vi "FTW-JSON-LexicalScan-Value.vi"(0 "JSON String":T1, 11 "error in":errorcluster) -> (4 "JSON String Out":T1, 8 "Container":variant, 15 "error out":errorcluster)   [LabVIEW 2015]
uses:
  FTW-JSON-LexicalScan.ctl
  container/FTW-Container.lvclass
panel:
  # "Inputs"
  # "Outputs"
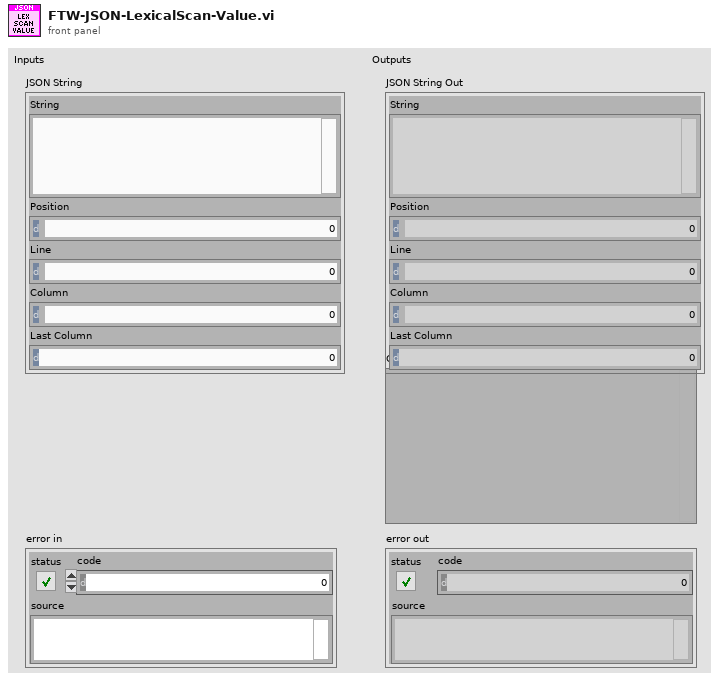
[diagram p1: front panel]
types:
  T1 = typedef "FTW-JSON-LexicalScan.ctl" = cluster{"String":string, "Position":i32, "Line":i32, "Column":i32, "Last Column":i32}
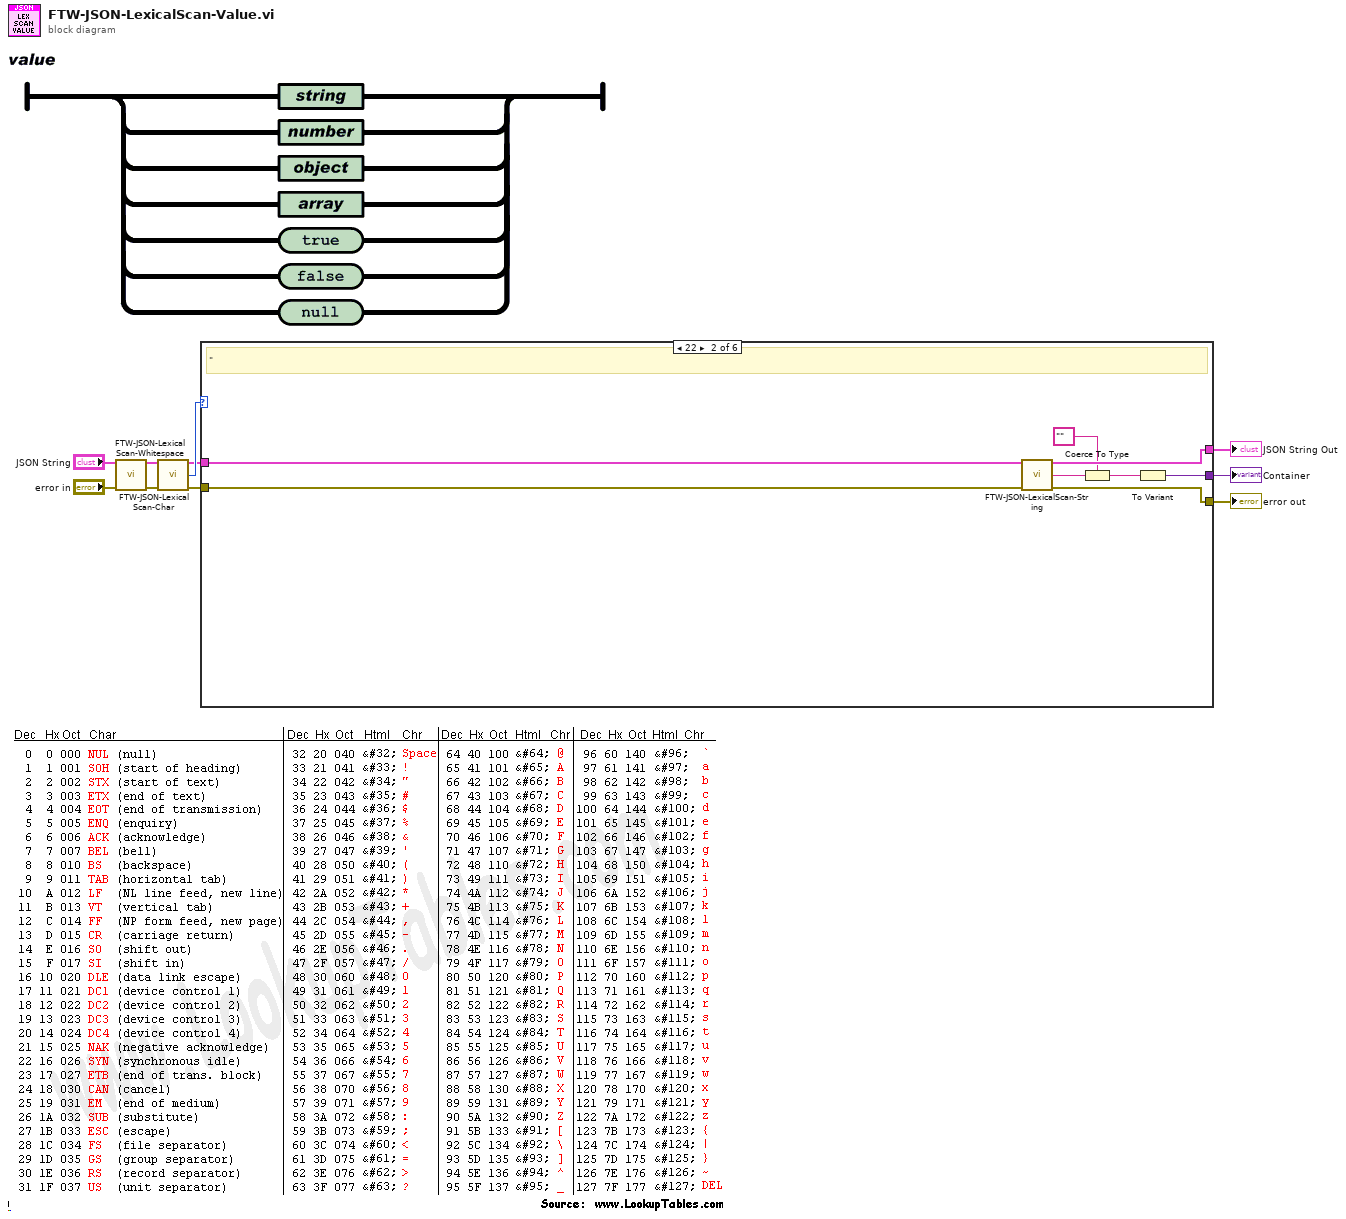
[diagram p0: block diagram]
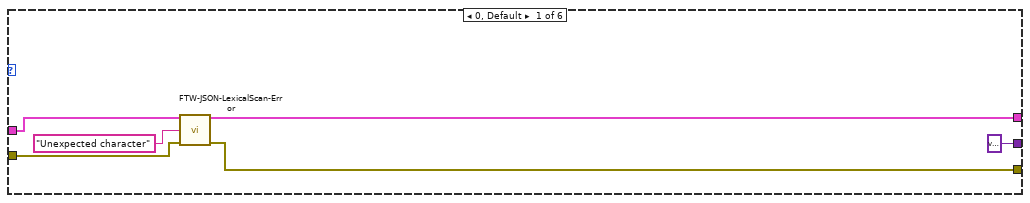
[diagram p2: hidden frame]
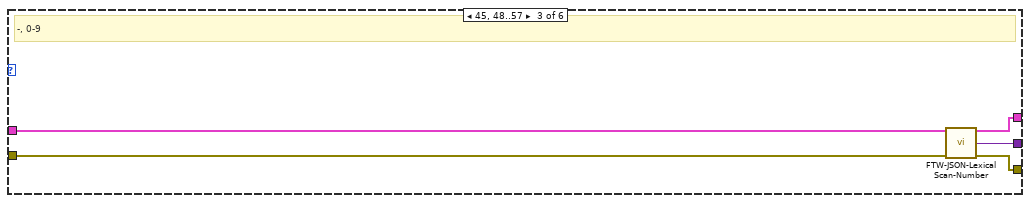
[diagram p3: hidden frame]
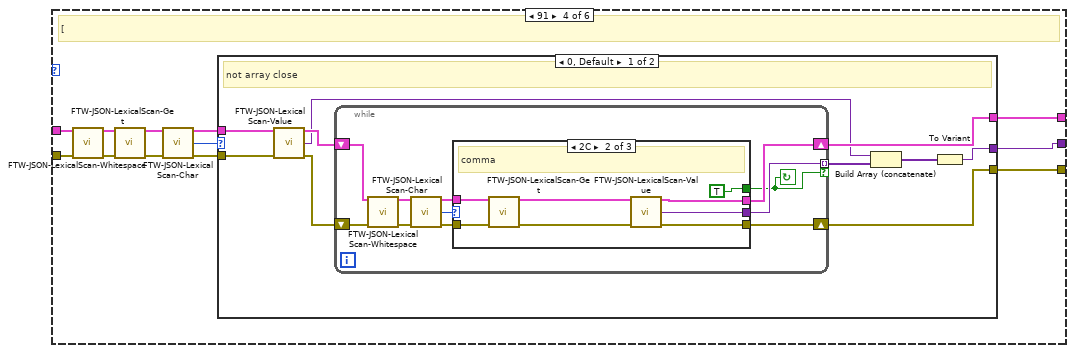
[diagram p4: hidden frame]
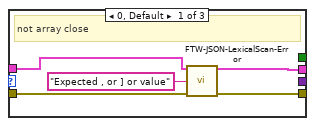
[diagram p5: hidden frame]
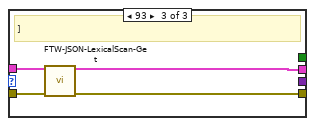
[diagram p6: hidden frame]
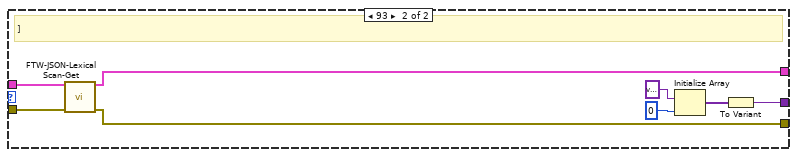
[diagram p7: hidden frame]
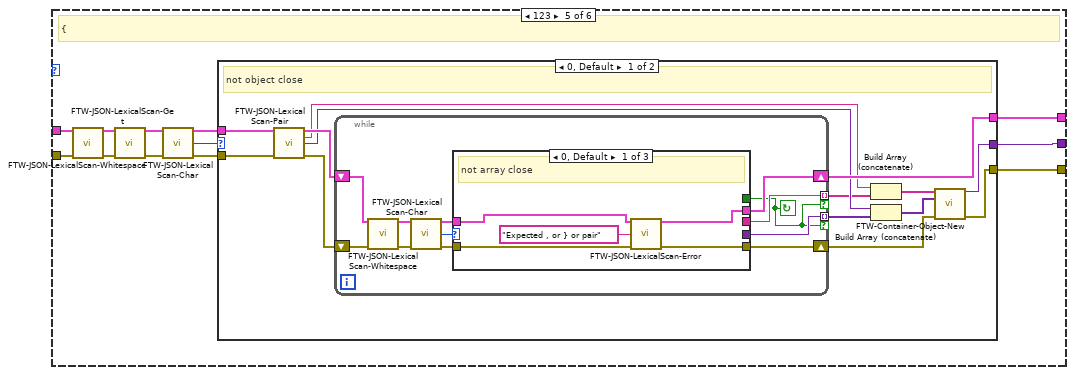
[diagram p8: hidden frame]
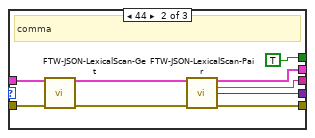
[diagram p9: hidden frame]
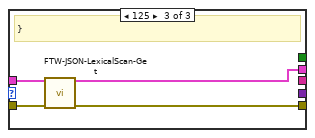
[diagram p10: hidden frame]
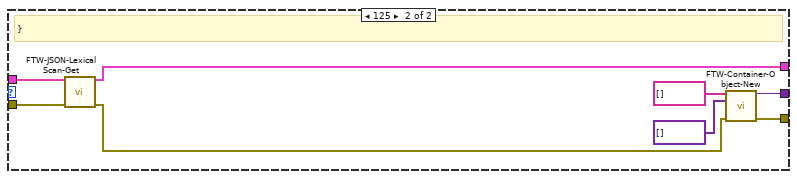
[diagram p11: hidden frame]
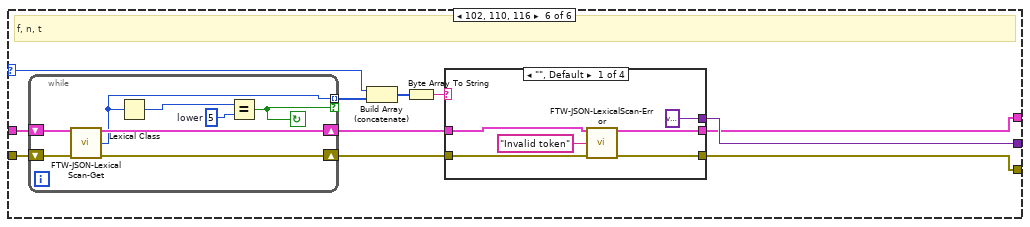
[diagram p12: hidden frame]
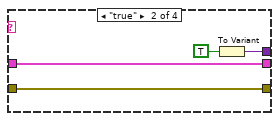
[diagram p13: hidden frame]
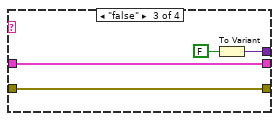
[diagram p14: hidden frame]
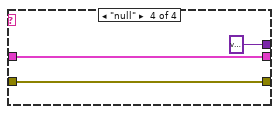
[diagram p15: hidden frame]
diagram:
  n1 = call "FTW-JSON-LexicalScan-Whitespace.vi"("JSON String"="JSON String", "error in"="error in") -> ("JSON String Out"=w1:T1, "error out"=w3:errorcluster)  [unwired: 12 in]
  n2 = call "FTW-JSON-LexicalScan-Char.vi"("JSON String"=w1, "error in"=w3) -> ("JSON String Out"=w7:T1, "Char"=w9:u8, "error out"=w8:errorcluster)  [unwired: 11 in]
  n3 = case shown="22" w9 {
    selector: w9 -> [_ _ _ _ _ w158]
    tunnel: w8 -> [w16 w23 w28 w41 w99 w161]
    tunnel: w7 -> [w13 w24 w29 w39 w97 w160]
    tunnel: [w14 w22 w27 w31 w89 w156] -> w6
    tunnel: [w12 w21 w26 w32 w90 w152] -> w5
    tunnel: [variant w19 w25 w30 w88 w154] -> w4
    frame 0, Default {
      n4 = call "FTW-JSON-LexicalScan-Error.vi"("JSON String"=w13, "Error String"="Unexpected character", "error in"=w16) -> ("JSON String Out"=w12:T1, "error out"=w14:errorcluster)  [unwired: 11 in]
    }
    frame 34 {
      # "\""
      n5 = call "FTW-JSON-LexicalScan-String.vi"("JSON String"=w24, "error in"=w23) -> ("JSON String Out"=w21:T1, "String"=w20:string, "error out"=w22:errorcluster)  [unwired: 10 in, 1 out]
      n6 = Coerce To Type(0:w20, 1:"") -> (2:w18:string)
      n7 = To Variant(anything=w18) -> (Variant=w19:variant)
    }
    frame 45, 48..57 {
      # "-, 0-9"
      n8 = call "FTW-JSON-LexicalScan-Number.vi"("JSON String"=w29, "error in"=w28) -> ("JSON String Out"=w26:T1, "Number"=w25:variant, "error out"=w27:errorcluster)  [unwired: 11 in]
    }
    frame 91 {
      # "["
      n9 = call "FTW-JSON-LexicalScan-Get.vi"("JSON String"=w39, "error in"=w41) -> ("JSON String Out"=w38:T1, "error out"=w40:errorcluster)  [unwired: 11 in, 1 out]
      n10 = call "FTW-JSON-LexicalScan-Whitespace.vi"("JSON String"=w38, "error in"=w40) -> ("JSON String Out"=w37:T1, "error out"=w36:errorcluster)  [unwired: 12 in]
      n11 = call "FTW-JSON-LexicalScan-Char.vi"("JSON String"=w37, "error in"=w36) -> ("JSON String Out"=w34:T1, "Char"=w35:u8, "error out"=w33:errorcluster)  [unwired: 11 in]
      n12 = case shown="0, Default" w35 {
        tunnel: w34 -> [w50 w81]
        tunnel: w33 -> [w51 w87]
        tunnel: [w46 w80] -> w32
        tunnel: [w47 w82] -> w31
        tunnel: [w42 w83] -> w30
        frame 0, Default {
          # "not array close"
          n13 = call "FTW-JSON-LexicalScan-Value.vi"("JSON String"=w50, "error in"=w51) -> ("JSON String Out"=w48:T1, "Container"=w44:variant, "error out"=w49:errorcluster)  [unwired: 11 in]
          n14 = while {
            shift-right: [w54] -> w47
            shift-left: w49 -> [w62]
            shift-right: [w55] -> w46
            shift-left: w48 -> [w60]
            tunnel: [w53] -> w45 mode=indexing if=w52
            stop <- w52 continue-if-true
            n15 = call "FTW-JSON-LexicalScan-Whitespace.vi"("JSON String"=w60, "error in"=w62) -> ("JSON String Out"=w59:T1, "error out"=w61:errorcluster)  [unwired: 12 in]
            n16 = call "FTW-JSON-LexicalScan-Char.vi"("JSON String"=w59, "error in"=w61) -> ("JSON String Out"=w58:T1, "Char"=w56:u8, "error out"=w57:errorcluster)  [unwired: 11 in]
            n17 = case shown="2C" w56 {
              tunnel: w58 -> [w65 w71 w77]
              tunnel: w57 -> [w67 w75 w79]
              tunnel: [w64 w73 w76] -> w55
              tunnel: [w66 w74 w78] -> w54
              tunnel: [_ w69 _] -> w53
              tunnel: [_ TRUE _] -> w52
              frame 0, Default {
                # "not array close"
                n18 = call "FTW-JSON-LexicalScan-Error.vi"("JSON String"=w65, "Error String"="Expected , or ] or value" ("Error Message"), "error in"=w67) -> ("JSON String Out"=w64:T1, "error out"=w66:errorcluster)  [unwired: 11 in]
              }
              frame 44 {
                # "comma"
                n19 = call "FTW-JSON-LexicalScan-Get.vi"("JSON String"=w71, "error in"=w75) -> ("JSON String Out"=w70:T1, "error out"=w72:errorcluster)  [unwired: 11 in, 1 out]
                n20 = call "FTW-JSON-LexicalScan-Value.vi"("JSON String"=w70, "error in"=w72) -> ("JSON String Out"=w73:T1, "Container"=w69:variant, "error out"=w74:errorcluster)  [unwired: 11 in]
              }
              frame 93 {
                # "]"
                n21 = call "FTW-JSON-LexicalScan-Get.vi"("JSON String"=w77, "error in"=w79) -> ("JSON String Out"=w76:T1, "error out"=w78:errorcluster)  [unwired: 11 in, 1 out]
              }
            }
          }
          n22 = Build Array (concatenate)(w44, w45) -> (w43:variant[])
          n23 = To Variant(anything=w43) -> (Variant=w42:variant)
        }
        frame 93 {
          # "]"
          n24 = call "FTW-JSON-LexicalScan-Get.vi"("JSON String"=w81, "error in"=w87) -> ("JSON String Out"=w80:T1, "error out"=w82:errorcluster)  [unwired: 11 in, 1 out]
          n25 = Initialize Array(variant, 0 ("dimension size")) -> (w84:variant[])
          n26 = To Variant(anything=w84) -> (Variant=w83:variant)
        }
      }
    }
    frame 123 {
      # "{"
      n27 = call "FTW-JSON-LexicalScan-Get.vi"("JSON String"=w97, "error in"=w99) -> ("JSON String Out"=w96:T1, "error out"=w98:errorcluster)  [unwired: 11 in, 1 out]
      n28 = call "FTW-JSON-LexicalScan-Whitespace.vi"("JSON String"=w96, "error in"=w98) -> ("JSON String Out"=w95:T1, "error out"=w94:errorcluster)  [unwired: 12 in]
      n29 = call "FTW-JSON-LexicalScan-Char.vi"("JSON String"=w95, "error in"=w94) -> ("JSON String Out"=w92:T1, "Char"=w93:u8, "error out"=w91:errorcluster)  [unwired: 11 in]
      n30 = case shown="0, Default" w93 {
        tunnel: w92 -> [w112 w145]
        tunnel: w91 -> [w113 w151]
        tunnel: [w108 w144] -> w90
        tunnel: [w105 w150] -> w89
        tunnel: [w104 w149] -> w88
        frame 0, Default {
          # "not object close"
          n31 = call "FTW-JSON-LexicalScan-Pair.vi"("JSON String"=w112, "error in"=w113) -> ("JSON String Out"=w110:T1, "Name"=w103:string, "Container"=w106:variant, "error out"=w111:errorcluster)  [unwired: 10 in]
          n32 = while {
            shift-right: [w117] -> w109
            shift-left: w111 -> [w125]
            shift-right: [w118] -> w108
            shift-left: w110 -> [w123]
            tunnel: [w116] -> w107 mode=indexing if=w114
            tunnel: [w115] -> w100 mode=indexing if=w114
            stop <- w114 continue-if-true
            n33 = call "FTW-JSON-LexicalScan-Whitespace.vi"("JSON String"=w123, "error in"=w125) -> ("JSON String Out"=w122:T1, "error out"=w124:errorcluster)  [unwired: 12 in]
            n34 = call "FTW-JSON-LexicalScan-Char.vi"("JSON String"=w122, "error in"=w124) -> ("JSON String Out"=w121:T1, "Char"=w119:u8, "error out"=w120:errorcluster)  [unwired: 11 in]
            n35 = case shown="0, Default" w119 {
              tunnel: w121 -> [w128 w135 w141]
              tunnel: w120 -> [w130 w139 w143]
              tunnel: [w127 w137 w140] -> w118
              tunnel: [w129 w138 w142] -> w117
              tunnel: [_ w133 _] -> w116
              tunnel: [_ TRUE _] -> w114
              tunnel: [_ w131 _] -> w115
              frame 0, Default {
                # "not array close"
                n36 = call "FTW-JSON-LexicalScan-Error.vi"("JSON String"=w128, "Error String"="Expected , or } or pair" ("Error Message"), "error in"=w130) -> ("JSON String Out"=w127:T1, "error out"=w129:errorcluster)  [unwired: 11 in]
              }
              frame 44 {
                # "comma"
                n37 = call "FTW-JSON-LexicalScan-Get.vi"("JSON String"=w135, "error in"=w139) -> ("JSON String Out"=w134:T1, "error out"=w136:errorcluster)  [unwired: 11 in, 1 out]
                n38 = call "FTW-JSON-LexicalScan-Pair.vi"("JSON String"=w134, "error in"=w136) -> ("JSON String Out"=w137:T1, "Name"=w131:string, "Container"=w133:variant, "error out"=w138:errorcluster)  [unwired: 10 in]
              }
              frame 125 {
                # "}"
                n39 = call "FTW-JSON-LexicalScan-Get.vi"("JSON String"=w141, "error in"=w143) -> ("JSON String Out"=w140:T1, "error out"=w142:errorcluster)  [unwired: 11 in, 1 out]
              }
            }
          }
          n40 = Build Array (concatenate)(w103, w100) -> (w102:string[])
          n41 = Build Array (concatenate)(w106, w107) -> (w101:variant[])
          n42 = call "FTW-Container-Object-New.vi"("Names"=w102, "Values"=w101, "error in"=w109) -> (4:w104:variant, "error out"=w105:errorcluster)  [unwired: 11 in]
        }
        frame 125 {
          # "}"
          n43 = call "FTW-JSON-LexicalScan-Get.vi"("JSON String"=w145, "error in"=w151) -> ("JSON String Out"=w144:T1, "error out"=w146:errorcluster)  [unwired: 11 in, 1 out]
          n44 = call "FTW-Container-Object-New.vi"("Names"=string[] [], "Values"=variant[] [], "error in"=w146) -> (4:w149:variant, "error out"=w150:errorcluster)  [unwired: 11 in]
        }
      }
    }
    frame 102, 110, 116 {
      # "f, n, t"
      n45 = while {
        shift-right: [w184] -> w153
        shift-left: w160 -> [w185]
        shift-right: [w186] -> w162
        shift-left: w161 -> [w187]
        tunnel: [w181] -> w159 mode=indexing if=w180
        stop <- w180 continue-if-true
        w182 = i16 5  # lower
        n46 = call "FTW-JSON-LexicalScan-Get.vi"("JSON String"=w185, "error in"=w187) -> ("JSON String Out"=w184:T1, "Char"=w181:u8, "error out"=w186:errorcluster)  [unwired: 11 in]
        n47 = Lexical Class(1:w181) -> (0:w183:i16)
        n48 = Equal?(x=w183, y=w182) -> (x = y?=w180:bool)
      }
      n49 = Build Array (concatenate)(w158, w159) -> (w157:u8[])
      n50 = Byte Array To String(unsigned byte array=w157) -> (string=w155:string)
      n51 = case shown="\"\", Default" w155 {
        tunnel: w162 -> [w168 w170 w174 w179]
        tunnel: [w166 w170 w174 w179] -> w156
        tunnel: [variant w171 w175 variant] -> w154
        tunnel: w153 -> [w165 w169 w173 w177]
        tunnel: [w163 w169 w173 w177] -> w152
        frame "", Default {
          n52 = call "FTW-JSON-LexicalScan-Error.vi"("JSON String"=w165, "Error String"="Invalid token" ("Error Message"), "error in"=w168) -> ("JSON String Out"=w163:T1, "error out"=w166:errorcluster)  [unwired: 11 in]
        }
        frame "true" {
          n53 = To Variant(anything=TRUE) -> (Variant=w171:variant)
        }
        frame "false" {
          n54 = To Variant(anything=FALSE) -> (Variant=w175:variant)
        }
        frame "null" {
        }
      }
    }
  }
  "Container" <- w4
  "error out" <- w6
  "JSON String Out" <- w5
